vi "Water Temperature Control.vi"() -> ()   [LabVIEW 2017]
uses:
  <vilib>/Instr/_visa.llb/VISA Configure Serial Port (Instr).vi
  <vilib>/addons/control/pid/pid.llb/PID (DBL).vi
  <vilib>/addons/control/pid/NI_PID_pid.lvlib
panel:
  in  "Control":bool=TRUE
  out "Actual DutyCycle":string
  in  "stop 2":bool
  in  "Write Delay":u32=1500
  out "Read Temperature":string
  in  "Multi Channel?":bool=TRUE
  in  "baud rate (9600) 2":u32=9600
  in  "Input Port / Port":refnum<visa-resource-name>="COM9"
  in  "baud rate (9600)":u32=9600
  in  "Read Delay":u32=100
  out "DutyCycle":string
  in  "stop":bool
  in  "PID gains":T1={"proportional gain (Kc)"=20.0, "integral time (Ti, min)"=0.01, "derivative time (Td, min)"=0.0} {"derivative time (Td, min)" format="%.3f"; "integral time (Ti, min)" format="%.3f"; "proportional gain (Kc)" format="%.3f"}
  in  "Suhu Air":dbl(slide)=30.0 scale=0.0..120.0
  out "Hasil":cluster{"Suhu Air":dbl, i32, i32}(graph)
  in  "Output Port":refnum<visa-resource-name>="COM4"
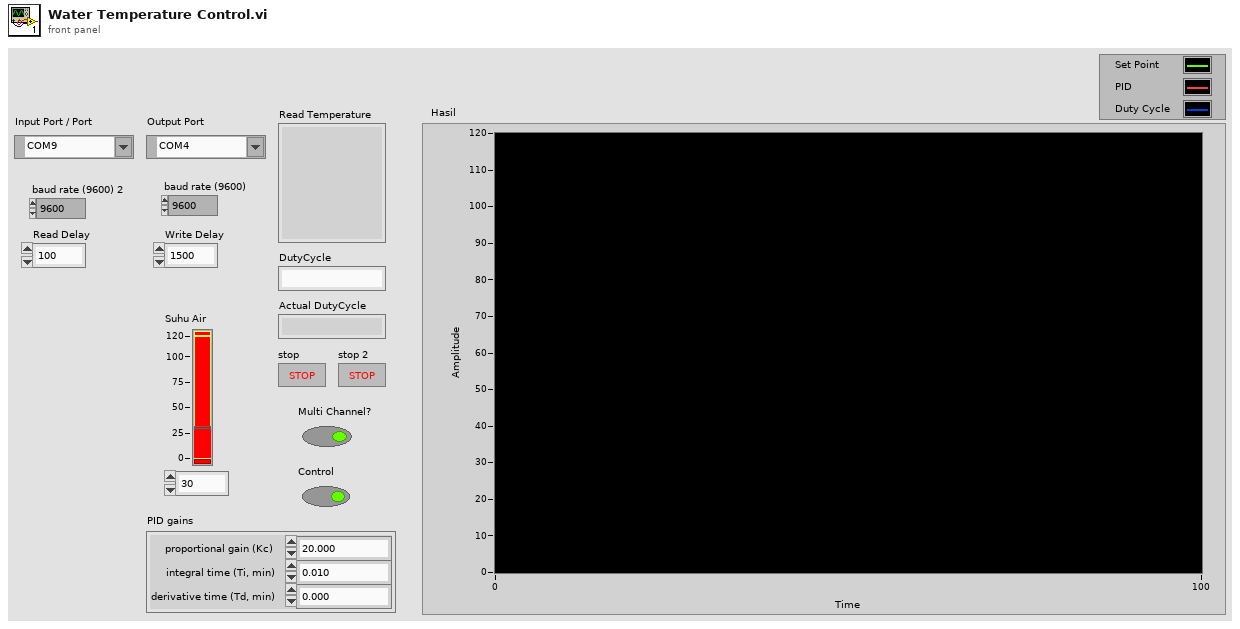
[diagram p1: front panel]
types:
  T1 = cluster{"proportional gain (Kc)":dbl, "integral time (Ti, min)":dbl, "derivative time (Td, min)":dbl}
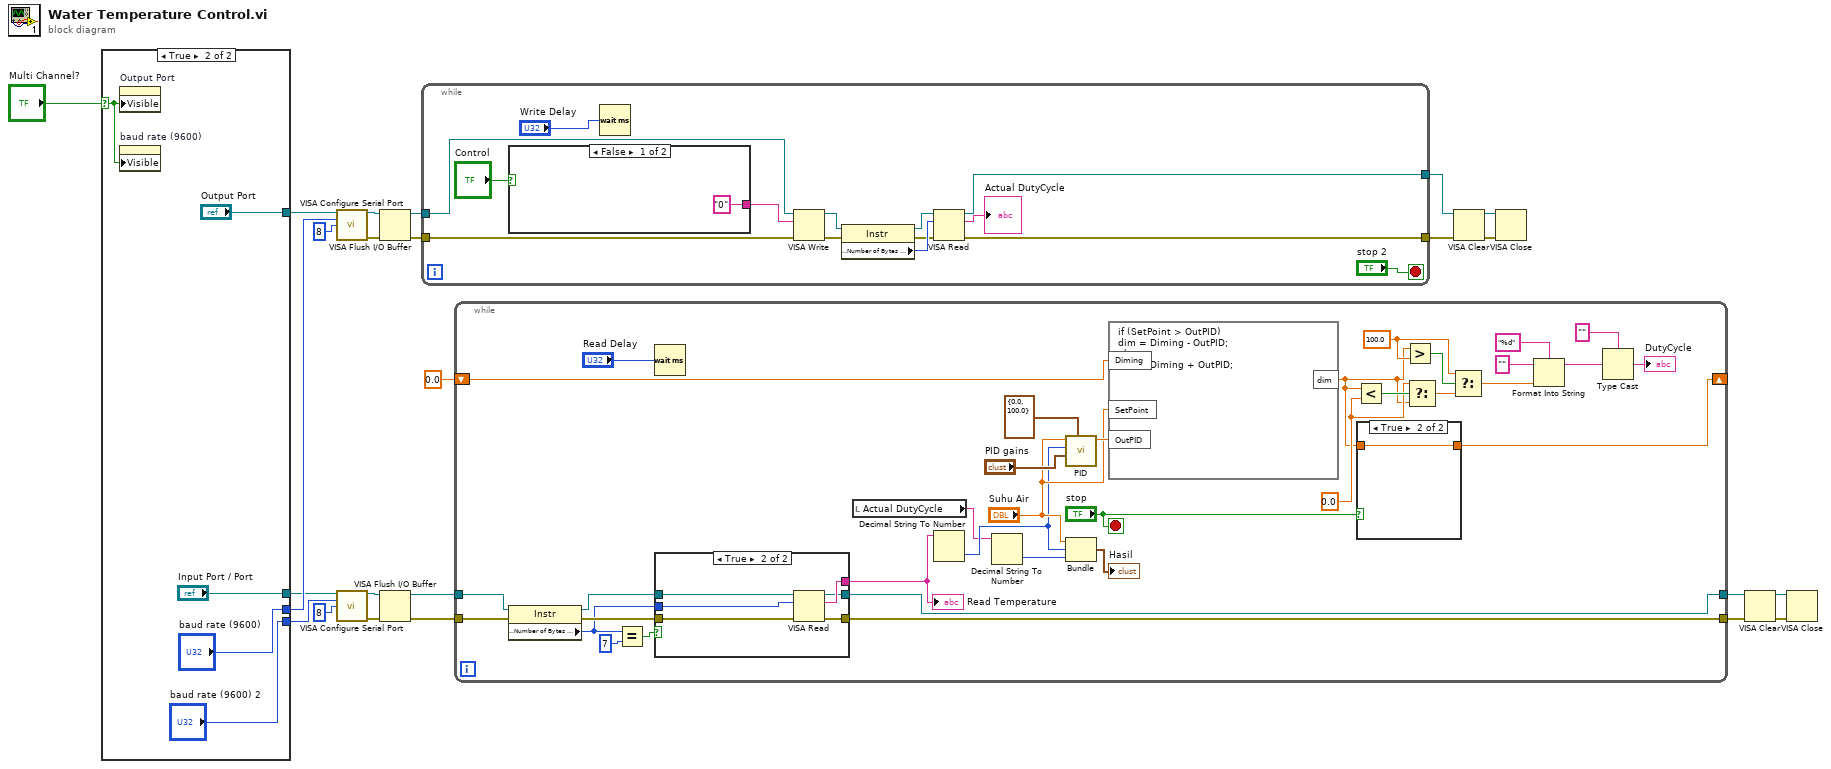
[diagram p0: block diagram]
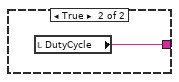
[diagram p2: hidden frame]
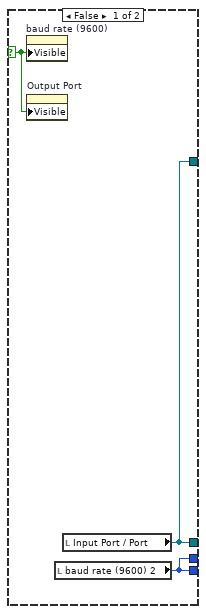
[diagram p3: hidden frame]
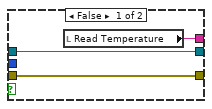
[diagram p4: hidden frame]
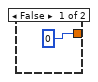
[diagram p5: hidden frame]
diagram:
  n1 = case shown="True" "Multi Channel?" {
    selector: "Multi Channel?" -> [w25 w28]
    tunnel: [w27 "Output Port"] -> w22
    tunnel: [w26 "baud rate (9600)"] -> w20
    tunnel: [w27 "Input Port / Port"] -> w16
    tunnel: [w26 "baud rate (9600) 2"] -> w15
    frame False {
      n2 = property on="baud rate (9600)" class="DigNum (strict)"("Visible"=w25) -> ()  [unwired: 2 in, 2 out]
      n3 = property on="Output Port" class="VISAName"("Visible"=w25) -> ()  [unwired: 2 in, 2 out]
      n4 = local read "baud rate (9600) 2"() -> (w26:u32)
      n5 = local read "Input Port / Port"() -> (w27:refnum<visa-resource-name>)
    }
    frame True {
      n6 = property on="Output Port" class="VISAName"("Visible"=w28) -> ()  [unwired: 2 in, 2 out]
      n7 = property on="baud rate (9600)" class="DigNum (strict)"("Visible"=w28) -> ()  [unwired: 2 in, 2 out]
    }
  }
  n8 = call-poly "VISA Configure Serial Port"("VISA resource name"=w22, "baud rate (9600)"=w20, "data bits (8)"=u16 8) -> ("VISA resource name out"=w18:refnum<visa-resource-name>, "error out"=w17:errorcluster)  [unwired: 11 in]
  n9 = call-poly "VISA Configure Serial Port"("VISA resource name"=w16, "baud rate (9600)"=w15, "data bits (8)"=u16 8) -> ("VISA resource name out"=w13:refnum<visa-resource-name>, "error out"=w12:errorcluster)  [unwired: 11 in]
  n10 = VISA Flush I/O Buffer(VISA resource name=w18, error in (no error)=w17) -> (VISA resource name out=w3:refnum<visa-resource-name>, error out=w4:errorcluster)  [unwired: 1 in]
  n11 = VISA Flush I/O Buffer(VISA resource name=w13, error in (no error)=w12) -> (VISA resource name out=w8:refnum<visa-resource-name>, error out=w7:errorcluster)  [unwired: 1 in]
  n12 = while {
    tunnel: w4 -> [w46]
    tunnel: w3 -> [w45]
    tunnel: [w41] -> w2
    tunnel: [w40] -> w1
    stop <- "stop 2" stop-if-true
    n13 = case shown="False" "Control" {
      tunnel: ["0" ("DutyCycle") w48] -> w44
      frame False {
      }
      frame True {
        n14 = local read "DutyCycle"() -> (w48:string)
      }
    }
    n15 = Wait (ms)(milliseconds to wait="Write Delay") -> ()  [unwired: 1 out]
    n16 = VISA Write(VISA resource name=w45, write buffer=w44, error in (no error)=w46) -> (VISA resource name out=w39:refnum<visa-resource-name>, error out=w38:errorcluster)  [unwired: 1 out]
    n17 = property class="Instr"(reference=w39, error in=w38) -> (reference out=w37:refnum<visa-resource-name>, error out=w35:errorcluster, "Serial Settings:Number of Bytes at Serial Port"=w36:u32)
    n18 = VISA Read(VISA resource name=w37, byte count=w36, error in (no error)=w35) -> (VISA resource name out=w41:refnum<visa-resource-name>, read buffer=→"Actual DutyCycle":string, error out=w40:errorcluster)  [unwired: 1 out]
  }
  n19 = while {
    shift-right: [w82] -> _
    shift-left: 0.0 -> [w79]
    tunnel: w8 -> [w61]
    tunnel: w7 -> [w60]
    tunnel: [w59] -> w6
    tunnel: [w58] -> w5
    stop <- "stop" stop-if-true
    w69 = 0.0 ("y")
    w70 = 100.0 ("y")
    n20 = property class="Instr"(reference=w61, error in=w60) -> (reference out=w56:refnum<visa-resource-name>, error out=w57:errorcluster, "Serial Settings:Number of Bytes at Serial Port"=w54:u32)
    n21 = Equal?(x=w54, y=u32 7) -> (x = y?=w52:bool)
    n22 = Wait (ms)(milliseconds to wait="Read Delay") -> ()  [unwired: 1 out]
    n23 = case shown="True" w52 {
      tunnel: [w85 w91] -> w59
      tunnel: [w83 w90] -> w51
      tunnel: [w84 w86] -> w58
      tunnel: w57 -> [w85 w89]
      tunnel: w56 -> [w84 w88]
      tunnel: w54 -> [_ w87]
      frame False {
        n24 = local read "Read Temperature"() -> (w83:string)
      }
      frame True {
        n25 = VISA Read(VISA resource name=w88, byte count=w87, error in (no error)=w89) -> (VISA resource name out=w86:refnum<visa-resource-name>, read buffer=w90:string, error out=w91:errorcluster)  [unwired: 1 out]
      }
    }
    "Read Temperature" <- w51
    n26 = local read "Actual DutyCycle"() -> (w50:string)
    n27 = Decimal String To Number(string=w51) -> (number=w73:i32)  [unwired: 2 in, 1 out]
    n28 = Decimal String To Number(string=w50) -> (number=w49:i32)  [unwired: 2 in, 1 out]
    n29 = call-poly <vilib>:"PID.vi"("output range"=cluster{"output high":dbl, "output low":dbl} {"output high"=0.0, "output low"=100.0}, "PID gains"="PID gains", "process variable"=w73, "setpoint"="Suhu Air") -> ("output"=w78:dbl)  [unwired: 6 in, 1 out]
    n30 = Bundle("Suhu Air"="Suhu Air", w73, w49) -> (→"Hasil":cluster{"Suhu Air":dbl, i32, i32})  [unwired: 1 in]
    n31 = formula code="if (SetPoint > OutPID)\ndim = Diming - OutPID;\nelse\ndim = Diming + OutPID;"("Diming"=w79, "SetPoint"="Suhu Air", "OutPID"=w78) -> ("dim"=w67:dbl)
    n32 = Less?(x=w67, y=w69) -> (x < y?=w71:bool)
    n33 = case shown="True" "stop" {
      tunnel: [0 w93] -> w82
      tunnel: w67 -> [_ w93]
      frame False {
      }
      frame True {
      }
    }
    n34 = Greater?(x=w67, y=w70) -> (0:w72:bool)
    n35 = Select(t=w69, s=w71, f=w67) -> (s? t:f=w68:dbl)
    n36 = Select(t=w70, s=w72, f=w68) -> (s? t:f=w66:dbl)
    n37 = Format Into String(format string="%d", initial string="", w66) -> (resulting string=w63:string)  [unwired: 1 in, 1 out]
    n38 = Type Cast(type="", x=w63) -> (*(type *) &x=→"DutyCycle":string)
  }
  n39 = VISA Clear(VISA resource name=w2, error in (no error)=w1) -> (VISA resource name out=w23:refnum<visa-resource-name>, error out=w24:errorcluster)
  n40 = VISA Close(VISA resource name=w23, error in (no error)=w24) -> ()  [unwired: 1 out]
  n41 = VISA Clear(VISA resource name=w5, error in (no error)=w6) -> (VISA resource name out=w10:refnum<visa-resource-name>, error out=w9:errorcluster)
  n42 = VISA Close(VISA resource name=w10, error in (no error)=w9) -> ()  [unwired: 1 out]
